vi "Initialize User Interface.vi"(8 "error in (no error)":errorcluster, 10 "Refnum":refnum<vi>, 11 "Sequencer in":refnum<class "Sequencer.lvclass">) -> (0 "error out":errorcluster, 3 "Sequencer out":refnum<class "Sequencer.lvclass">)   [LabVIEW 2024, in "Ramses Sequencer.lvlib" / "Sequencer.lvclass"]
uses:
  Sequencer.lvclass
  Base Step/Base Step.lvclass/Base Step.ctl
  <vilib>/Utility/miscctls.llb/LVRowAndColumnTypeDef.ctl
  Sequence/Sequence.lvclass
  Base Step/Base Step.lvclass
  Sequencer.lvclass/Sequencer.ctl
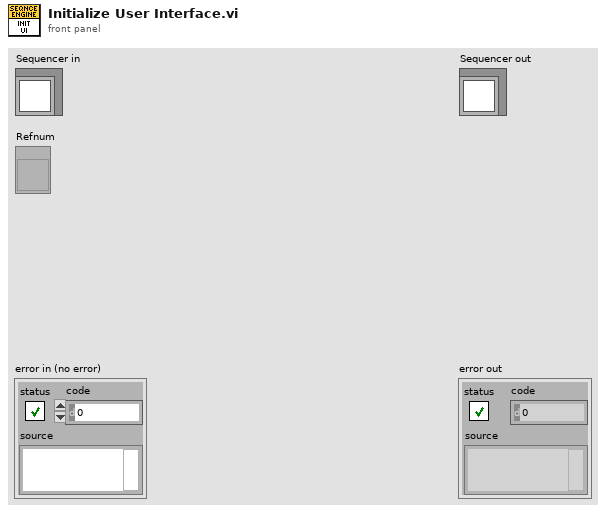
[diagram p1: front panel]
types:
  T1 = typedef "LVRowAndColumnTypeDef.ctl" = cluster{"Row":i32, "Column":i32}
  T2 = typedef "Ramses Sequencer.lvlib/Base Step.lvclass/Step State.ctl" = cluster{"Result":string, "Status":string, "Enabled":bool, "Upper":string, "Target":string, "Lower":string, "Value":string}
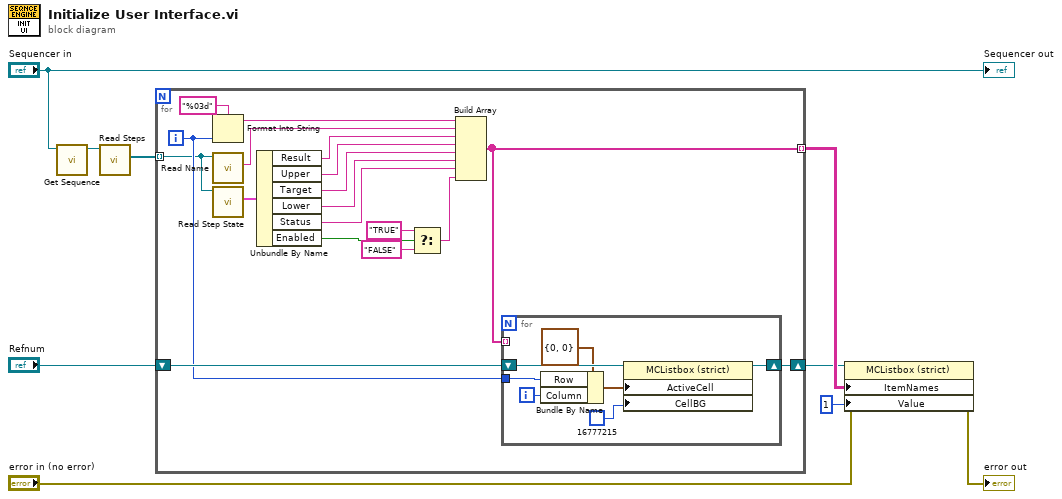
[diagram p0: block diagram]
diagram:
  n1 = call "Get Sequence.vi"("Sequencer in"="Sequencer in") -> ("Sequence"=w9:refnum<class "Sequence.lvclass">)  [unwired: 9 in, 1 out]
  n2 = call-dynamic "Read Steps.vi"("Sequence in"=w9) -> ("Steps"=w8:refnum<class "Base Step.lvclass">[])  [unwired: 8 in, 2 out]
  n3 = for {
    tunnel: w8 -> [w11] mode=indexing
    tunnel: [w13] -> w7 mode=indexing
    shift-right: [w14] -> w1
    shift-left: "Refnum" -> [w15]
    i -> [w12]
    n4 = Format Into String(format string="%03d", w12) -> (resulting string=w26:string)  [unwired: 2 in, 1 out]
    n5 = call-dynamic "Read Name.vi"("Base Step in"=w11) -> ("Name"=w25:string)  [unwired: 8 in, 2 out]
    n6 = call "Read Step State.vi"("Base Step in"=w11) -> ("Step State"=w10:T2)  [unwired: 8 in, 2 out]
    n7 = Unbundle By Name(w10) -> ("Result"=w24:string, "Upper"=w23:string, "Target"=w22:string, "Lower"=w21:string, "Status"=w20:string, "Enabled"=w18:bool)
    n8 = Select(t="TRUE" ("format string"), s=w18, f="FALSE" ("format string")) -> (s? t:f=w16:string)
    n9 = Build Array(w26, w25, w24, w23, w22, w21, w20, w16) -> (w13:string[])
    n10 = for {
      shift-right: [w33] -> w14
      shift-left: w15 -> [w34]
      tunnel: w12 -> [w30]
      tunnel: w13 -> [_] mode=indexing
      i -> [w29]
      n11 = Bundle By Name(cluster=T1 {"Row"=0, "Column"=0} ("Active Cell:Active Cell"), "Row"=w30, "Column"=w29) -> (w31:T1)
      n12 = property class="MCListbox (strict)"(reference=w34, "ActiveCell"=w31, "CellBG"=u32 16777215 ("Color")) -> (reference out=w33:refnum<vi>)  [unwired: 1 in, 1 out]
    }
  }
  n13 = property class="MCListbox (strict)"(reference=w1, error in="error in (no error)", "ItemNames"=w7, "Value"=1) -> (error out=→"error out":errorcluster)  [unwired: 1 out]
  "Sequencer out" <- "Sequencer in"
